vi "Clean up Node-Child Maps.vi"(7 "AtomicSet":refnum<class "DBSet.lvclass">, 11 "Raw Source to Sink Array":T1) -> (3 "Cleaned Source to Sink Array":T1)   [LabVIEW 2020]
uses:
  DBSet/DBSet.lvclass
  Node.ctl
  Source to Sink Array.ctl
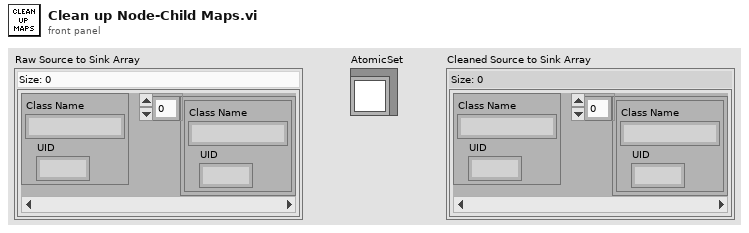
[diagram p1: front panel]
types:
  T1 = typedef "Source to Sink Array.ctl" = map{T2, T2[]}
  T2 = typedef "Node.ctl" = cluster{"Class Name":string, "UID":i32}
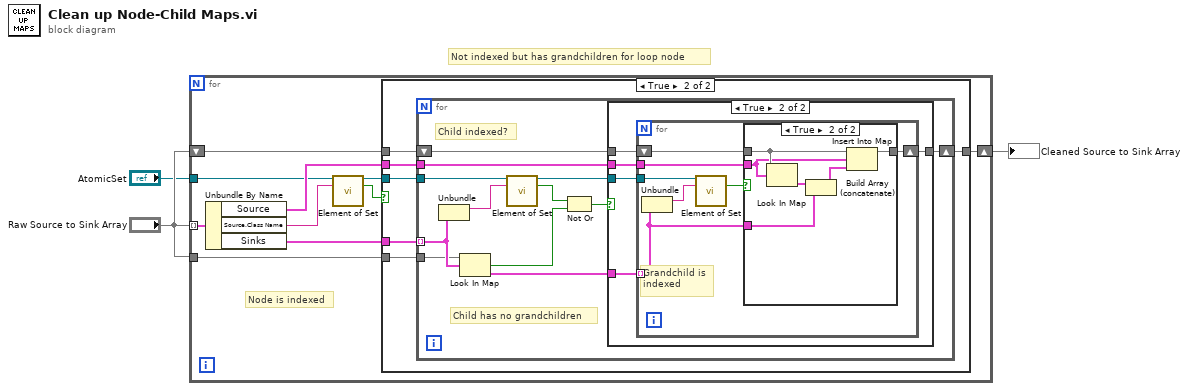
[diagram p0: block diagram]
diagram:
  # "Not indexed but has grandchildren for loop node"
  n1 = for {
    tunnel: "Raw Source to Sink Array" -> [w13] mode=indexing
    shift-right: [w8] -> w2
    shift-left: "Raw Source to Sink Array" -> [w11]
    tunnel: "AtomicSet" -> [w7]
    tunnel: "Raw Source to Sink Array" -> [w9]
    # "Node is indexed"
    n2 = Unbundle By Name(w13) -> ("Source"=w10:T2, "Source.Class Name"=w6:string, "Sinks"=w12:T2[])
    n3 = call "Element of Set.vi"("DBSet in"=w7, "Element"=w6) -> ("DBSet out"=w4:refnum<class "DBSet.lvclass">, "Found?"=w5:bool)  [unwired: 11 in, 1 out]
    n4 = case shown="True" w5 {
      tunnel: w12 -> [_ w18]
      tunnel: w4 -> [_ w20]
      tunnel: w11 -> [w14 w19]
      tunnel: w10 -> [_ w15]
      tunnel: w9 -> [_ w17]
      tunnel: [w14 w16] -> w8
      frame False {
      }
      frame True {
        n5 = for {
          tunnel: w18 -> [w32] mode=indexing
          tunnel: w20 -> [w24]
          shift-right: [w26] -> w16
          shift-left: w19 -> [w28]
          tunnel: w17 -> [w27]
          tunnel: w15 -> [w25]
          # "Child has no grandchildren"
          # "Child indexed?"
          n6 = Unbundle(w32) -> ("Class Name"=w22:string)  [unwired: 1 out]
          n7 = Look In Map(map=w27, key=w32) -> (key not found?=w30:bool, value=w29:T2[])  [unwired: 1 in]
          n8 = call "Element of Set.vi"("DBSet in"=w24, "Element"=w22) -> ("DBSet out"=w23:refnum<class "DBSet.lvclass">, "Found?"=w21:bool)  [unwired: 11 in, 1 out]
          n9 = Not Or(1:w30, 2:w21) -> (0:w31:bool)
          n10 = case shown="True" w31 {
            tunnel: w29 -> [_ w38]
            tunnel: w23 -> [_ w37]
            tunnel: w28 -> [w33 w36]
            tunnel: [w33 w35] -> w26
            tunnel: w25 -> [_ w34]
            frame False {
            }
            frame True {
              n11 = for {
                tunnel: w38 -> [w42] mode=indexing
                tunnel: w37 -> [w41]
                shift-right: [w44] -> w35
                shift-left: w36 -> [w45]
                tunnel: w34 -> [w43]
                # "Grandchild is\nindexed"
                n12 = Unbundle(w42) -> ("Class Name"=w40:string)  [unwired: 1 out]
                n13 = call "Element of Set.vi"("DBSet in"=w41, "Element"=w40) -> ("Found?"=w39:bool)  [unwired: 11 in, 2 out]
                n14 = case shown="True" w39 {
                  tunnel: w45 -> [w46 w52]
                  tunnel: [w46 w51] -> w44
                  tunnel: w43 -> [_ w47]
                  tunnel: w42 -> [_ w49]
                  frame False {
                  }
                  frame True {
                    n15 = Look In Map(map=w52, key=w47) -> (value=w50:T2[])  [unwired: 1 in, 1 out]
                    n16 = Build Array (concatenate)(w50, w49) -> (w48:T2[])
                    n17 = Insert Into Map(map in=w52, key=w47, value=w48) -> (map out=w51:T1)  [unwired: 2 out]
                  }
                }
              }
            }
          }
        }
      }
    }
  }
  "Cleaned Source to Sink Array" <- w2
